vi "DAQ Init_Multiple.vi"(0 "Model":string) -> (1 "task out":refnum<k21>, 2 "Task_Switch":refnum<k21>, 3 "error out":errorcluster)   [LabVIEW 2023]
uses:
  <vilib>/DAQmx/create/channels.llb/DAQmx Create Channel (DO-Digital Output).vi
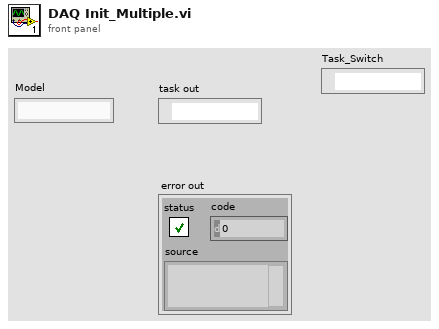
[diagram p1: front panel]
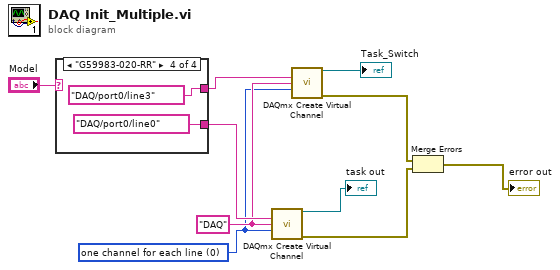
[diagram p0: block diagram]
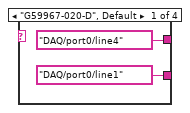
[diagram p2: hidden frame]
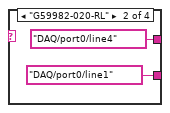
[diagram p3: hidden frame]
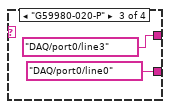
[diagram p4: hidden frame]
diagram:
  w3 = "DAQ" ("name to assign")
  w2 = 0 items=["one channel for each line", "one channel for all lines"] ("line grouping")
  n1 = case shown="\"G59983-020-RR\"" "Model" {
    tunnel: [tag "DAQ/port0/line1" ("lines") tag "DAQ/port0/line1" ("lines") tag "DAQ/port0/line0" ("lines") tag "DAQ/port0/line0" ("lines")] -> w9
    tunnel: [tag "DAQ/port0/line4" ("lines") tag "DAQ/port0/line4" ("lines") tag "DAQ/port0/line3" ("lines") tag "DAQ/port0/line3" ("lines")] -> w1
    frame "G59967-020-D", Default {
    }
    frame "G59982-020-RL" {
    }
    frame "G59980-020-P" {
    }
    frame "G59983-020-RR" {
    }
  }
  n2 = call-poly <vilib>:"DAQmx Create Virtual Channel.vi"("lines"=w9, "name to assign"=w3, "line grouping"=w2) -> ("task out"=→"task out":refnum<k21>, "error out"=w6:errorcluster)  [unwired: 11 in]
  n3 = call-poly <vilib>:"DAQmx Create Virtual Channel.vi"("lines"=w1, "name to assign"=w3, "line grouping"=w2) -> ("task out"=→"Task_Switch":refnum<k21>, "error out"=w5:errorcluster)  [unwired: 11 in]
  n4 = Merge Errors(w5, w6) -> (→"error out":errorcluster)
